vi "number_to_string.vi"(11 "input 1":ext) -> (3 "String":string)   [LabVIEW 2019]
panel:
  out "error out":errorcluster
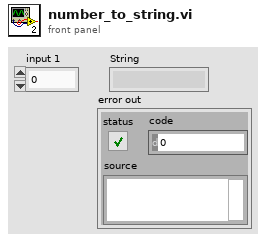
[diagram p1: front panel]
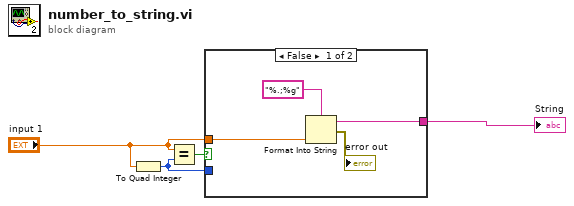
[diagram p0: block diagram]
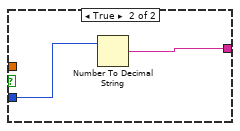
[diagram p2: hidden frame]
diagram:
  n1 = To Quad Integer(1:"input 1") -> (0:w3:i64)
  n2 = Equal?(x="input 1", y=w3) -> (x = y?=w1:bool)
  n3 = case shown="False" w1 {
    tunnel: "input 1" -> [w7 _]
    tunnel: w3 -> [_ w10]
    tunnel: [w6 w9] -> w4
    frame False {
      n4 = Format Into String(format string="%.;%g", w7) -> (resulting string=w6:string, error out=→"error out":errorcluster)  [unwired: 2 in]
    }
    frame True {
      n5 = Number To Decimal String(number=w10) -> (decimal integer string=w9:string)  [unwired: 1 in]
    }
  }
  "String" <- w4
